vi "get Front Panel control references.vi"(8 "error in (no error)":errorcluster, 11 "Main VI":refnum<vi>) -> (0 "error out":errorcluster)   [LabVIEW 2012]
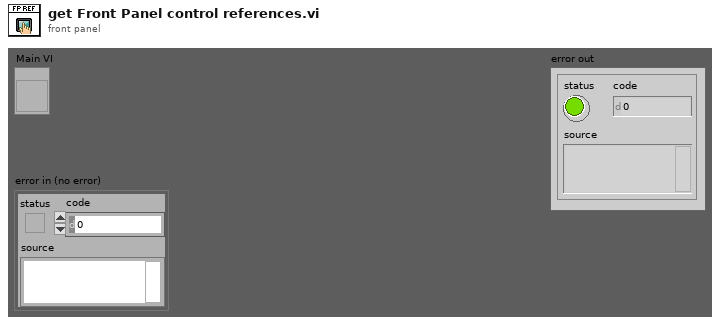
[diagram p1: front panel]
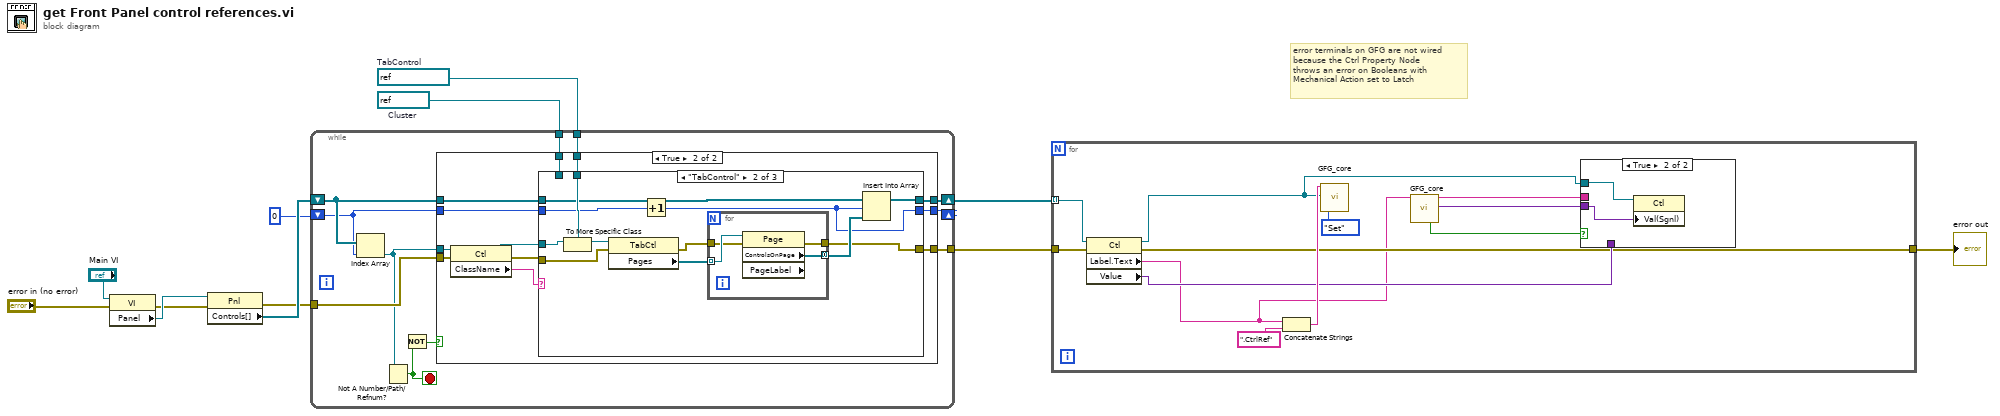
[diagram p0: block diagram]
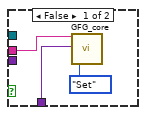
[diagram p2: hidden frame]
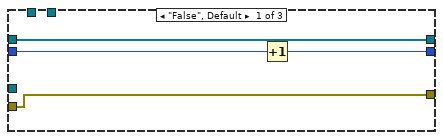
[diagram p4: hidden frame]
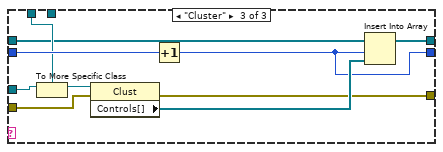
[diagram p5: hidden frame]
diagram:
  w3 = refnum<vi> refnum  # Cluster
  w10 = refnum<vi> refnum  # TabControl
  # "error terminals on GFG are not wired\nbecause the Ctrl Property Node\nthrows an error on Booleans with\nMechanical Action set to Latch"
  n1 = property class="VI"(reference="Main VI", error in="error in (no error)") -> (error out=w8:errorcluster, "Panel"=w12:refnum<vi>)  [unwired: 1 out]
  n2 = property class="Pnl"(reference=w12, error in=w8) -> (error out=w7:errorcluster, "Controls[]"=w11:refnum<vi>[])  [unwired: 1 out]
  n3 = while {
    shift-right: [w21] -> w6
    shift-left: w11 -> [w22]
    tunnel: w10 -> [w23]
    shift-right: [w19] -> _
    shift-left: 0 -> [w20]
    tunnel: w7 -> [w18]
    tunnel: w3 -> [w17]
    tunnel: [w14] -> w2
    stop <- w15 stop-if-true
    n4 = Index Array(array=w22, index=w20) -> (element=w13:refnum<vi>)
    n5 = Not A Number/Path/Refnum?(number/path/refnum=w13) -> (NaN/Path/Refnum?=w15:bool)
    n6 = Not(x=w15) -> (.not. x?=w16:bool)
    n7 = case shown="True" w16 {
      tunnel: w23 -> [_ w37]
      tunnel: w22 -> [w26 w36]
      tunnel: [w26 w35] -> w21
      tunnel: w20 -> [w25 w34]
      tunnel: [w25 w33] -> w19
      tunnel: w18 -> [w24 w32]
      tunnel: w17 -> [_ w30]
      tunnel: [w24 w29] -> w14
      tunnel: w13 -> [_ w28]
      frame False {
      }
      frame True {
        n8 = property class="Ctl"(reference=w28, error in=w32) -> (reference out=w38:refnum<vi>, error out=w31:errorcluster, "ClassName"=w27:string)
        n9 = case shown="\"TabControl\"" w27 {
          tunnel: w38 -> [_ w54 w68]
          tunnel: w37 -> [_ w53 _]
          tunnel: w36 -> [w42 w44 w60]
          tunnel: [w42 w49 w66] -> w35
          tunnel: w34 -> [w41 w45 w64]
          tunnel: [w40 w43 w59] -> w33
          tunnel: w31 -> [w39 w48 w65]
          tunnel: [w39 w46 w61] -> w29
          tunnel: w30 -> [_ _ w63]
          frame "False", Default {
            n10 = Increment(x=w41) -> (x+1=w40:i32)
          }
          frame "TabControl" {
            n11 = To More Specific Class(target class=w53, reference=w54) -> (specific class reference=w52:refnum<vi>)  [unwired: 1 in, 1 out]
            n12 = property class="TabCtl"(reference=w52, error in=w48) -> (error out=w47:errorcluster, "Pages"=w51:refnum<vi>[])  [unwired: 1 out]
            n13 = Increment(x=w45) -> (x+1=w43:i32)
            n14 = for {
              tunnel: w51 -> [w58] mode=indexing
              tunnel: [w57] -> w50 mode=concatenating
              tunnel: w47 -> [w56]
              tunnel: [w55] -> w46
              n15 = property class="Page" props=["ControlsOnPage", "PageLabel"](reference=w58, error in=w56) -> (error out=w55:errorcluster, "ControlsOnPage"=w57:refnum<vi>[])  [unwired: 2 out]
            }
            n16 = Insert Into Array(array=w44, index=w43, new element=w50) -> (w49:refnum<vi>[])
          }
          frame "Cluster" {
            n17 = To More Specific Class(target class=w63, reference=w68) -> (specific class reference=w67:refnum<vi>)  [unwired: 1 in, 1 out]
            n18 = property class="Clust"(reference=w67, error in=w65) -> (error out=w61:errorcluster, "Controls[]"=w62:refnum<vi>[])  [unwired: 1 out]
            n19 = Increment(x=w64) -> (x+1=w59:i32)
            n20 = Insert Into Array(array=w60, index=w59, new element=w62) -> (w66:refnum<vi>[])
          }
        }
      }
    }
  }
  n21 = for {
    tunnel: w6 -> [w77] mode=indexing
    tunnel: w2 -> [w79]
    tunnel: [w74] -> w1
    n22 = property class="Ctl"(reference=w77, error in=w79) -> (reference out=w69:refnum<vi>, error out=w74:errorcluster, "Label.Text"=w72:string, "Value"=w76:variant)
    n23 = Concatenate Strings(w72, ".CtrlRef" ("string")) -> (w78:string)
    n24 = call "GFG_core.vi"("Variable Name in"=w78, "Variant in"=w69, "Action"=enum16{"Init", "Set", "Get"}."Set") -> ()  [unwired: 10 in, 7 out]
    n25 = call "GFG_core.vi"("Variable Name in"=w72) -> ("Found/Replaced"=w73:bool, "Variable Name Out"=w71:string, "Variant Out"=w70:variant)  [unwired: 12 in, 4 out]
    n26 = case shown="True" w73 {
      tunnel: w76 -> [w83 _]
      tunnel: w71 -> [w81 _]
      tunnel: w70 -> [_ w84]
      tunnel: w69 -> [_ w85]
      frame False {
        n27 = call "GFG_core.vi"("Variable Name in"=w81, "Variant in"=w83, "Action"=enum16{"Init", "Set", "Get"}."Set") -> ()  [unwired: 10 in, 7 out]
      }
      frame True {
        n28 = property class="Ctl"(reference=w85, "Val(Sgnl)"=w84) -> ()  [unwired: 1 in, 2 out]
      }
    }
  }
  "error out" <- w1
